vi "Write Camera Name.vi"(8 "error in (no error)":errorcluster, 10 "IMAQdx Session":T1, 11 "HIJ Vision Camera App Dialog in":refnum<class "HIJ Vision Camera App Dialog.lvclass">) -> (0 "error out":errorcluster, 3 "HIJ Vision Camera App Dialog out":refnum<class "HIJ Vision Camera App Dialog.lvclass">)   [LabVIEW 2020, in "HIJ Vision Camera App Dialog.lvlib" / "HIJ Vision Camera App Dialog.lvclass"]
uses:
  HIJ Vision Camera App Dialog.lvclass
  HIJ Vision Camera App Dialog.lvclass/HIJ Vision Camera App Dialog.ctl
  <vilib>/userdefined/High Color/IMAQdx.ctl
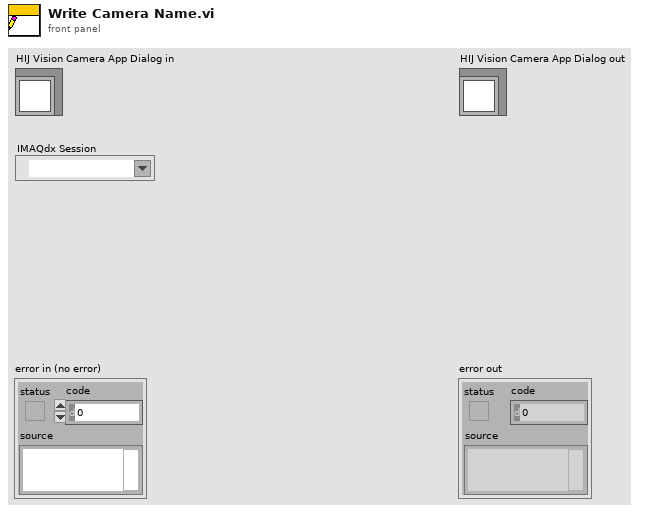
[diagram p1: front panel]
types:
  T1 = typedef "IMAQdx.ctl" = refnum<k21>
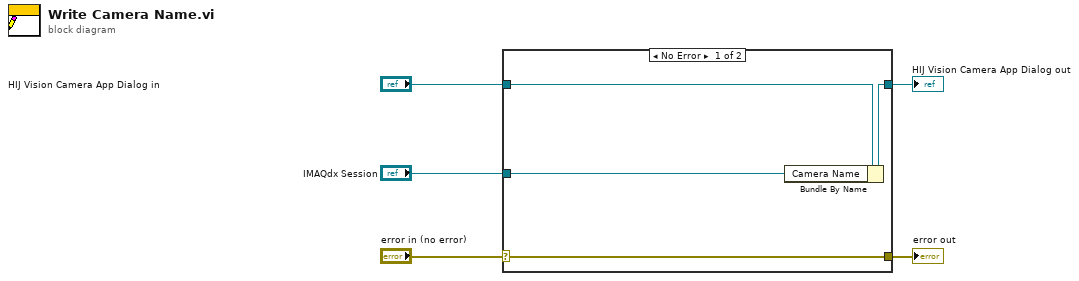
[diagram p0: block diagram]
diagram:
  n1 = case shown="No Error" "error in (no error)" {
    selector: "error in (no error)" -> [w9 w10]
    tunnel: [w9 w10] -> w4
    tunnel: [w7 w11] -> w2
    tunnel: "HIJ Vision Camera App Dialog in" -> [w8 w11]
    tunnel: "IMAQdx Session" -> [w6 _]
    frame No Error {
      n2 = Bundle By Name(cluster=w8, "Camera Name"=w6) -> (w7:refnum<class "HIJ Vision Camera App Dialog.lvclass">)
    }
    frame Error {
    }
  }
  "error out" <- w4
  "HIJ Vision Camera App Dialog out" <- w2
